vi "Zero Phase Filter (CDB).vi"(9 "Forward Coefficients":dbl[](array[numeric]), 10 "Reverse Coefficients":dbl[](array[numeric]), 11 "X":cdb[](array[numeric])) -> (0 "error":i32, 3 "Filtered X":cdb[](array[numeric]))   [LabVIEW 2017, in "NI_AALBase.lvlib"]
doc: "Applies a zero phase filter to an input sequence <B>X</B>. Wire data to the <B>X</B> input to determine the polymorphic instance to use or manually select the instance."
uses:
  <vilib>/Analysis/NI_AALBase.lvlib
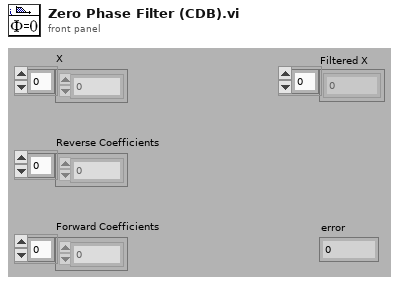
[diagram p1: front panel]
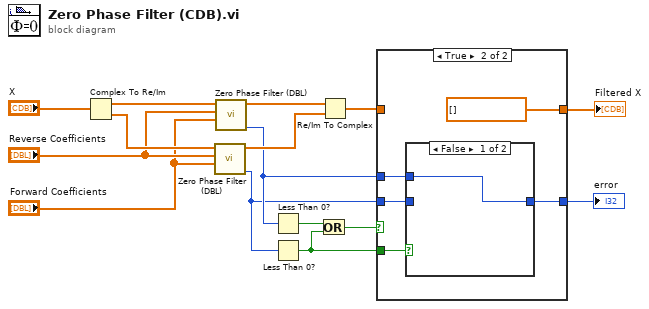
[diagram p0: block diagram]
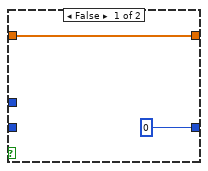
[diagram p2: hidden frame]
diagram:
  n1 = Complex To Re/Im(x + iy="X") -> (x=w14:dbl[], y=w13:dbl[])
  n2 = call <vilib>:"Zero Phase Filter (DBL).vi"("Forward Coefficients"="Forward Coefficients", "Reverse Coefficients"="Reverse Coefficients", "X"=w13) -> ("error"=w6:i32, "Filtered X"=w10:dbl[])  [unwired: 7 in]
  n3 = call <vilib>:"Zero Phase Filter (DBL).vi"("Forward Coefficients"="Forward Coefficients", "Reverse Coefficients"="Reverse Coefficients", "X"=w14) -> ("error"=w7:i32, "Filtered X"=w11:dbl[])  [unwired: 7 in]
  n4 = Less Than 0?(x=w7) -> (x < 0?=w12:bool)
  n5 = Less Than 0?(x=w6) -> (x < 0?=w3:bool)
  n6 = Or(x=w12, y=w3) -> (x .or. y?=w4:bool)
  n7 = Re/Im To Complex(1:w10, 2:w11) -> (0:w9:cdb[])
  n8 = case shown="True" w4 {
    tunnel: w9 -> [w17 _]
    tunnel: w3 -> [_ w22]
    tunnel: w6 -> [_ w21]
    tunnel: w7 -> [_ w20]
    tunnel: [0 ("error") w19] -> w5
    tunnel: [w17 cdb[] []] -> w8
    frame False {
    }
    frame True {
      n9 = case shown="False" w22 {
        tunnel: [w23 w24] -> w19
        tunnel: w21 -> [_ w24]
        tunnel: w20 -> [w23 _]
        frame False {
        }
        frame True {
        }
      }
    }
  }
  "Filtered X" <- w8
  "error" <- w5
